vi "subVI_CFO_savetotext_USRP.vi"(8 "RSSI":dbl, 11 "file path (dialog if empty)":path) -> ()   [LabVIEW 2021]
uses:
  <vilib>/Utility/file.llb/Write Delimited Spreadsheet (DBL).vi
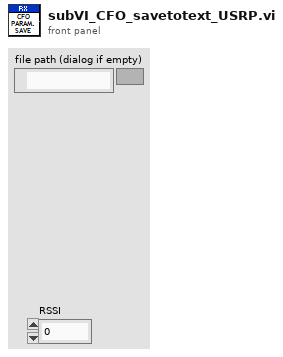
[diagram p1: front panel]
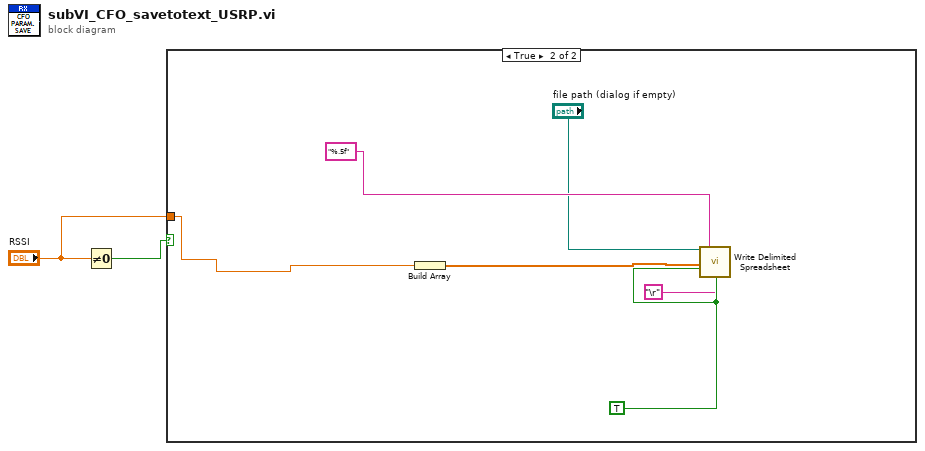
[diagram p0: block diagram]
diagram:
  n1 = Not Equal To 0?(x="RSSI") -> (x != 0?=w2:bool)
  n2 = case shown="True" w2 {
    tunnel: "RSSI" -> [_ w3]
    frame False {
    }
    frame True {
      w7 = TRUE ("transpose? (no:F)")
      n3 = Build Array(w3) -> (w4:dbl[])
      n4 = call-poly <vilib>:"Write Delimited Spreadsheet.vi"("file path (dialog if empty)"="file path (dialog if empty)", "format (%.3f)"="%.5f", "1D data"=w4, "append to file? (new file:F)"=w7, "transpose? (no:F)"=w7, "delimiter (\\t)"="\r") -> ()  [unwired: 8 in, 2 out]
    }
  }
